vi "ExSubSetRGB.vi"(3 "error in (no error)":errorcluster, 4 "Adjustments":T1={"Type of Bayer"=1, "Red Gain"=1.0, "Green Gain"=1.0, "Blue Gain"=1.0, "Bit shift"=0, "Red Offset"=0.0, "Green Offset"=0.0, "Blue Offset"=0.0} {"Blue Offset" format="%.2f"; "Green Offset" format="%.2f"; "Red Offset" format="%.2f"; "Blue Gain" format="%.2f"; "Green Gain" format="%.2f"; "Red Gain" format="%.2f"; "Type of Bayer" max=4 step=1}, 5 "RGB Handle":u32, 6 "Image handle":u32) -> (0 "error out":errorcluster, 1 "RGB handle":u32, 2 "Image handle":u32)   [LabVIEW 2012]
panel:
  # "ExSubSetRGB.vi : this subvi sets the RGB parameters\nand generates an RGB image from a normal bayer image"
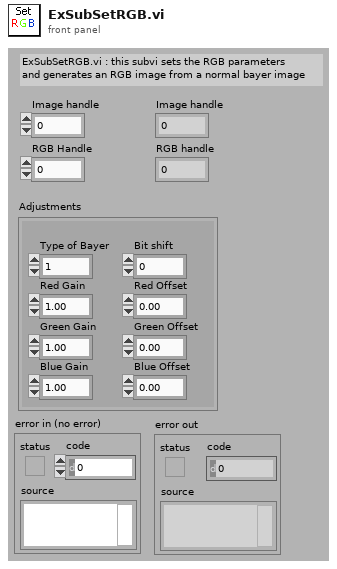
[diagram p1: front panel]
types:
  T1 = cluster{"Type of Bayer":u32, "Red Gain":dbl, "Green Gain":dbl, "Blue Gain":dbl, "Bit shift":u16, "Red Offset":dbl, "Green Offset":dbl, "Blue Offset":dbl}
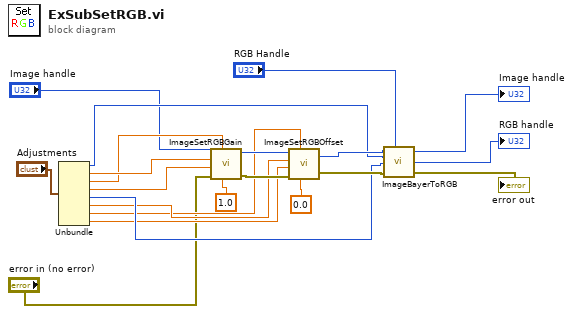
[diagram p0: block diagram]
diagram:
  n1 = Unbundle("Adjustments") -> ("Type of Bayer"=w13:u32, "Red Gain"=w11:dbl, "Green Gain"=w9:dbl, "Blue Gain"=w10:dbl, "Bit shift"=w12:u16, "Red Offset"=w8:dbl, "Green Offset"=w6:dbl, "Blue Offset"=w7:dbl)
  n2 = call <userlib>:"ImageSetRGBGain.vi"("reserved"=1.0, "Green Gain"=w9, "error in (no error)"="error in (no error)", "Blue Gain"=w10, "Red Gain"=w11, "Image Handle"="Image handle") -> ("error out"=w20:errorcluster, "Image Handle"=w21:u32)
  n3 = call <userlib>:"ImageSetRGBOffset.vi"("reserved"=0.0, "Green Offset"=w6, "error in (no error)"=w20, "Blue Offset"=w7, "Red Offset"=w8, "Image Handle"=w21) -> ("error out"=w17:errorcluster, "Image Handle"=w15:u32)
  n4 = call <userlib>:"ImageBayerToRGB.vi"("Image Handle"=w15, "Type of Bayer"=w13, "Shift amount"=w12, "error in"=w17, "RGB Handle In"="RGB Handle") -> ("Image Handle"=→"Image handle":u32, "RGB Image Handle"=→"RGB handle":u32, "error out"=→"error out":errorcluster)
